vi "Counter with Race Condition.vi"() -> ()   [LabVIEW 2014]
panel:
  out "Running Total":i32
  in  "Stop Button":bool
  out "Loop Count Difference":i32
  out "Loop Count 2":i32
  out "Loop Count 1":i32
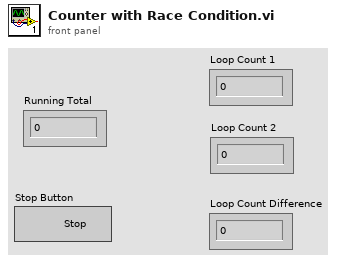
[diagram p1: front panel]
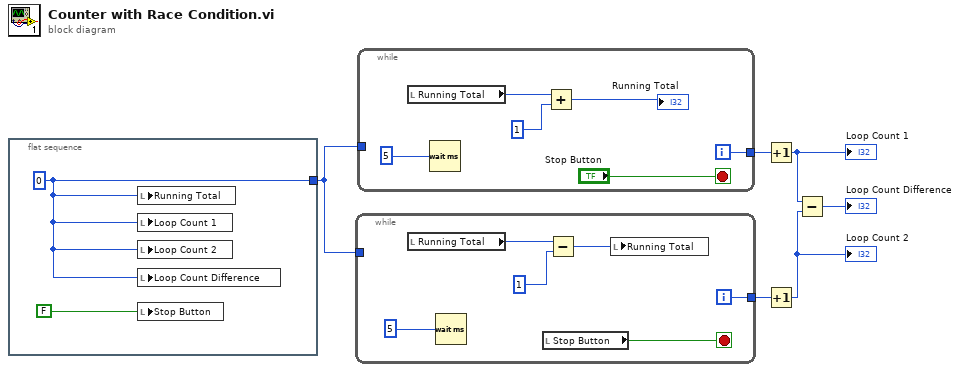
[diagram p0: block diagram]
diagram:
  n1 = flat-sequence {
    tunnel: [w7] -> w4
    frame #0 {
      w7 = 0 ("Running Total")
      n2 = local write "Running Total"(w7) -> ()
      n3 = local write "Loop Count 1"(w7) -> ()
      n4 = local write "Loop Count 2"(w7) -> ()
      n5 = local write "Loop Count Difference"(w7) -> ()
      n6 = local write "Stop Button"(FALSE ("Stop Button")) -> ()
    }
  }
  n7 = while {
    tunnel: [w12] -> w5
    tunnel: w4 -> [_]
    i -> [w12]
    stop <- w14 stop-if-true
    n8 = local read "Running Total"() -> (w11:i32)
    n9 = Wait (ms)(milliseconds to wait=u32 5) -> ()  [unwired: 1 out]
    n10 = local read "Stop Button"() -> (w14:bool)
    n11 = Subtract(x=w11, y=1 ("x")) -> (x-y=w9:i32)
    n12 = local write "Running Total"(w9) -> ()
  }
  n13 = while {
    tunnel: [w16] -> w6
    tunnel: w4 -> [_]
    i -> [w16]
    stop <- "Stop Button" stop-if-true
    n14 = local read "Running Total"() -> (w17:i32)
    n15 = Wait (ms)(milliseconds to wait=u32 5) -> ()  [unwired: 1 out]
    n16 = Add(x=w17, y=1 ("x")) -> (x+y=→"Running Total":i32)
  }
  n17 = Increment(x=w6) -> (x+1=w3:i32)
  "Loop Count 1" <- w3
  n18 = Increment(x=w5) -> (x+1=w2:i32)
  "Loop Count 2" <- w2
  n19 = Subtract(x=w3, y=w2) -> (x-y=→"Loop Count Difference":i32)
